vi "Low Pass Filter.vi"(8 "error in (no error)":errorcluster, 10 "Signal []":waveform(dbl)[](array[waveform]), 11 "Lockin.DAQ":refnum<class "Lockin.DAQ.lvclass">) -> (0 "error out":errorcluster, 1 "Fc (Hz)":dbl, 2 "Filtered Signal []":waveform(dbl)[](array[waveform]), 3 "Lockin.DAQ":refnum<class "Lockin.DAQ.lvclass">)   [LabVIEW 2016, in "Lockin.DAQ.lvclass"]
uses:
  Lockin.DAQ.lvclass
  Lockin.DAQ.lvclass/Lockin.DAQ.ctl
  <vilib>/addons/Digital Filter Design/Process.llb/DFD Filtering (Wfm NChan).vi
  <vilib>/addons/Digital Filter Design/NI_DigFilterLicensed.lvlib
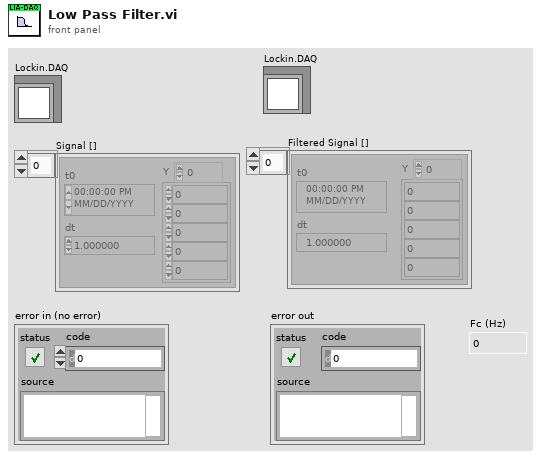
[diagram p1: front panel]
types:
  T1 = enum16{"Lowpass", "Highpass", "Bandpass", "Bandstop"}
  T2 = typedef "NI_DigFilterLicensed.lvlib/DFD Filter Obj.ctl" = cluster{"mSRate_Fs":dbl, "mSRate_Version":string, "mSRate_Comments":string, "mSRate_OrgCoef":T3, "mSRate_CurCoef":T3, "mSRate_Quantized?":bool, "mSRate_QCoef":T3, "mSRate_QSettings":T5[], "mSRate_Order":i32, "mSRate_Scaling":cluster{"mSRate_ScaleByPowerOf2?":bool, "mSRate_ScaleType":T7}}
  T3 = typedef "NI_DigFilterLicensed.lvlib/DFD Filter Coef.ctl" = cluster{"type":T4, "gain":dbl, "coef a (k)":dbl[], "coef b (v)":dbl[]}
  T4 = typedef "NI_DigFilterLicensed.lvlib/DFD Filter Structure Type Selector.ctl" = enum16{"Undefined", "FIR Direct Form", "FIR Direct Form Transposed", "FIR Symmetric", "FIR Antisymmetric", "IIR Direct Form I", "IIR Direct Form I Transposed", "IIR Direct Form II", "IIR Direct Form II Transposed", "IIR Cascaded Second Order Sections Form I", "IIR Cascaded Second Order Sections Form I Transposed", "IIR Cascaded Second Order Sections Form II", "IIR Cascaded Second Order Sections Form II Transposed", "Lattice Allpass (basic sections)", "Lattice Allpass (one multiplier sections)", "Lattice Allpass (normalized sections)", "Lattice AR (basic sections)", "Lattice AR (one multiplier sections)", "Lattice AR (normalized sections)", "Lattice MA (minimum phase)", "Lattice MA (maximum phase)", "Lattice ARMA (basic sections)", "Lattice ARMA (one multiplier sections)", "Lattice ARMA (normalized sections)"}
  T5 = typedef "NI_DigFilterLicensed.lvlib/dfd_Internal Quantization Settings.ctl" = cluster{"source":T6, "wl":i16, "iwl":i16, "overflow mode":enum16{"Saturation", "Wrap"}, "rounding mode":enum16{"Nearest", "Truncation"}, "signed?":bool}
  T6 = typedef "NI_DigFilterLicensed.lvlib/dfd_Internal Quantization Srcs.ctl" = u16
  T7 = typedef "NI_DigFilterLicensed.lvlib/DFD Coef Norm Type.ctl" = enum16{"No Norm", "Time Domain 1-Norm", "Time Domain 2-Norm", "Time Domain Inf-Norm"}
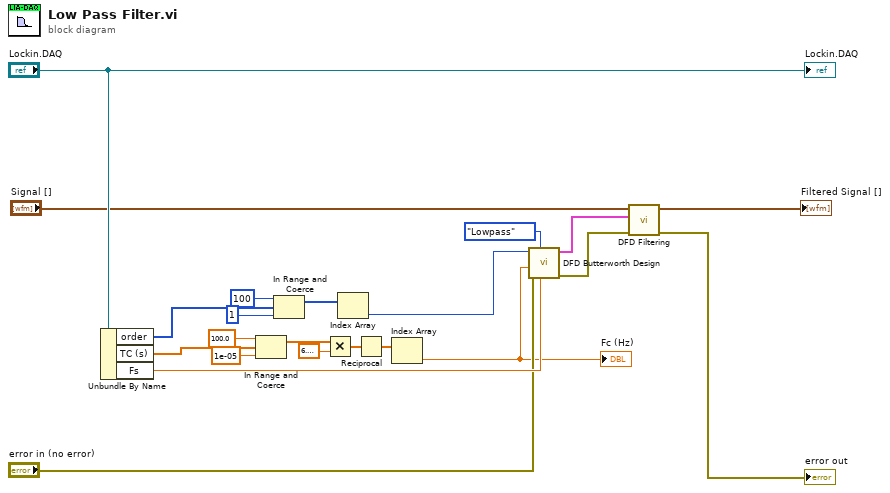
[diagram p0: block diagram]
diagram:
  n1 = Unbundle By Name("Lockin.DAQ") -> ("order"=w19:i32[], "TC (s)"=w20:dbl[], "Fs"=w18:dbl)
  n2 = In Range and Coerce(upper limit=100.0, x=w20, lower limit=1e-05) -> (coerced(x)=w7:dbl[])  [unwired: 1 out]
  n3 = In Range and Coerce(upper limit=100, x=w19, lower limit=1) -> (coerced(x)=w11:i32[])  [unwired: 1 out]
  n4 = Multiply(x=w7, y=6.283185307179586) -> (x*y=w3:dbl[])
  n5 = Index Array(array=w11) -> (element=w21:i32)  [unwired: 1 in]
  n6 = Reciprocal(x=w3) -> (1/x=w12:dbl[])
  n7 = Index Array(array=w12) -> (element=w14:dbl)  [unwired: 1 in]
  "Fc (Hz)" <- w14
  n8 = call <vilib>:"DFD Butterworth Design.vi"("fs [Hz]"=w18, "filter type"=T1."Lowpass", "error in (no error)"="error in (no error)", "low cutoff freq [Hz]"=w14, "order"=w21) -> ("error out"=w17:errorcluster, "filter out"=w13:T2)  [unwired: 5 in]
  n9 = call-poly <vilib>:"DFD Filtering.vi"("error in (no error)"=w17, "filter"=w13, "signal in"="Signal []") -> ("error out"=→"error out":errorcluster, "signal out"=→"Filtered Signal []":waveform(dbl)[])  [unwired: 7 in]
  "Lockin.DAQ" <- "Lockin.DAQ"
